vi "ActTurn.vi"(9 "FirstTime":bool, 10 "MaxSpeed (Deg/s)":dbl, 11 "Degrees":dbl) -> (0 "RotationSpeedDemand Deg/Sec":dbl, 3 "Done":bool)   [LabVIEW 2023]
doc: "Robot will turn a set number of degrees utilizing position control \n\nInputs:\n-- MaxSpeed -- Double -- In ft/s, the MaxSpeed the robot can go -- \n-- Degrees -- Double -- Rotation in degrees you want the robot to go -- \n-- FirstTime -- Boolean -- Input true the first time this function is called, sets the target position -- \n\nOutputs:\n-- Done -- Bool -- has the robot reached its target distance -- \n-- LeftSpeedDemand -- Double -- Speed Demand for left drive train inorder to reach target -- \n-- RightSpeedDemand -- Double -- Speed Demand for left drive train inorder to reach target --"
uses:
  <vilib>/Rock Robotics/WPI/ThirdParty/JAS_Junk/TrajLib/SlewRateLimiter_New.vi
  <vilib>/Rock Robotics/WPI/ThirdParty/JAS_Junk/TrajLib/SlewRateLimiter_Reset.vi
  <vilib>/Rock Robotics/WPI/ThirdParty/JAS_Junk/TrajLib/SlewRateLimiter_Calculate.vi
  <vilib>/Rock Robotics/WPI/ThirdParty/JAS_Junk/TrajLib/SlewRateLimiter_SetRate.vi
  <vilib>/Rock Robotics/WPI/ThirdParty/JAS_Junk/TrajLib/Util_GetTime.vi
  <vilib>/Rock Robotics/WPI/ThirdParty/JAS_Junk/TrajLib/VI/Util_GetTime_U32.vi
  <vilib>/Rock Robotics/Network Tables/NT Write Number.vi
  <vilib>/Rock Robotics/WPI/ThirdParty/JAS_Junk/TrajLib/VI/Util_GetTime_U64.vi
  <vilib>/Rock Robotics/Network Tables/NT Write Boolean.vi
  <vilib>/Rock Robotics/WPI/ThirdParty/JAS_Junk/TrajLib/Trajectory_Library.lvlib
panel:
  out "Unfiltetred Done":bool
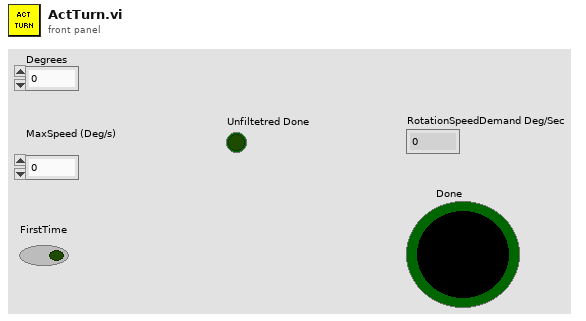
[diagram p1: front panel]
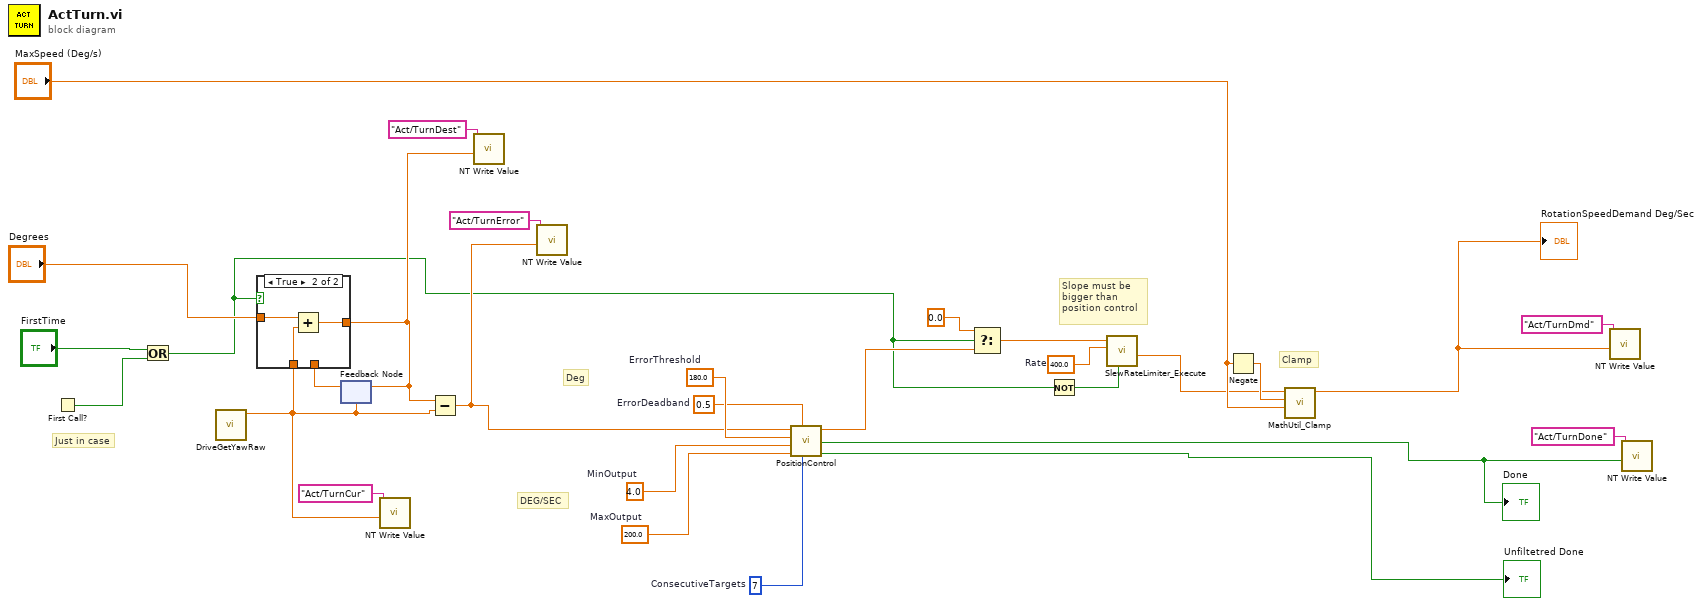
[diagram p0: block diagram]
diagram:
  w7 = 400.0  # Rate
  w21 = 200.0  # MaxOutput
  w22 = 4.0  # MinOutput
  w25 = 7  # ConsecutiveTargets
  w26 = 0.5  # ErrorDeadband
  w27 = 180.0  # ErrorThreshold
  # "Deg"
  # "DEG/SEC"
  # "Slope must be\nbigger than\nposition control"
  # "Just in case"
  # "Clamp"
  n1 = First Call?() -> (First Call?: T/F=w9:bool)
  n2 = Or(x="FirstTime", y=w9) -> (x .or. y?=w1:bool)
  n3 = call "DriveGetYawRaw.vi"() -> ("YawRaw"=w11:dbl)  [unwired: 11 in]
  n4 = feedback #1(w11) -> (w28:dbl)
  n5 = case shown="True" w1 {
    tunnel: "Degrees" -> [_ w33]
    tunnel: [w30 w32] -> w13
    tunnel: w28 -> [w30 _]
    tunnel: w11 -> [_ w31]
    frame False {
    }
    frame True {
      n6 = Add(x=w33, y=w31) -> (x+y=w32:dbl)
    }
  }
  n7 = feedback-in #1(w13) -> ()
  n8 = call-poly <vilib>:"NT Write Value.vi"("value"=w11, "name"="Act/TurnCur") -> ()  [unwired: 9 in, 1 out]
  n9 = Subtract(x=w13, y=w11) -> (x-y=w18:dbl)
  n10 = call-poly <vilib>:"NT Write Value.vi"("value"=w13, "name"="Act/TurnDest") -> ()  [unwired: 9 in, 1 out]
  n11 = call-poly <vilib>:"NT Write Value.vi"("value"=w18, "name"="Act/TurnError") -> ()  [unwired: 9 in, 1 out]
  n12 = call "PositionControl.vi"("ConsecutiveTargets"=w25, "ErrorDeadband"=w26, "MaxOutput"=w21, "MinOutput"=w22, "ErrorThreshold"=w27, "Error"=w18) -> ("UnfilteredOnTarget"=→"Unfiltetred Done":bool, "OnTarget"=w16:bool, "OutputValue"=w3:dbl)  [unwired: 3 in]
  "Done" <- w16
  n13 = Select(t=0.0, s=w1, f=w3) -> (s? t:f=w5:dbl)
  n14 = Not(x=w1) -> (.not. x?=w4:bool)
  n15 = call <vilib>:"SlewRateLimiter_Execute.vi"("Enable"=w4, "PositiveRate"=w7, "Input"=w5) -> ("Output"=w2:dbl)  [unwired: 7 in, 1 out]
  n16 = Negate(x="MaxSpeed (Deg/s)") -> (-x=w24:dbl)
  n17 = call <vilib>:"MathUtil_Clamp.vi"("High Limit"="MaxSpeed (Deg/s)", "Low Limit"=w24, "Value"=w2) -> ("Result"=w8:dbl)  [unwired: 8 in]
  "RotationSpeedDemand Deg/Sec" <- w8
  n18 = call-poly <vilib>:"NT Write Value.vi"("value"=w8, "name"="Act/TurnDmd") -> ()  [unwired: 9 in, 1 out]
  n19 = call-poly <vilib>:"NT Write Value.vi"("value"=w16, "name"="Act/TurnDone") -> ()  [unwired: 9 in, 1 out]
